vi "Config Power Sequence.vi"(7 "Get/Update":enum16{"Get Seq", "Update Seq"}(ring), 8 "Error In":errorcluster, 10 "Power Seq":T1 {"Duration" format="%<%H:%M:%S>t"}, 11 "Seq file path":path=path "C:/Users/skkjh/OneDrive - Chroma ATE/Working Copy/Cobra Single/NI-9651 SoM RT/RT_Configuration file/Cobra Extra Settings.ini") -> (0 "Error Out":errorcluster, 2 "Power Seq out":T1 {"Duration" format="%<%H:%M:%S>t"}, 3 "Seq path out":path)   [LabVIEW 2019, in "GUI.lvlib"]
uses:
  GUI.lvlib
  Controls/Profile Sequence.ctl
  <vilib>/Utility/config.llb/Read Key (I32).vi
  <vilib>/Utility/config.llb/Read Key (U32).vi
  <vilib>/Utility/config.llb/Read Key (String).vi
  <vilib>/Utility/config.llb/Write Key (String).vi
  <vilib>/Utility/config.llb/Write Key (I32).vi
  <vilib>/Utility/config.llb/Write Key (Double).vi
  <vilib>/Utility/config.llb/NI_LVConfig.lvlib
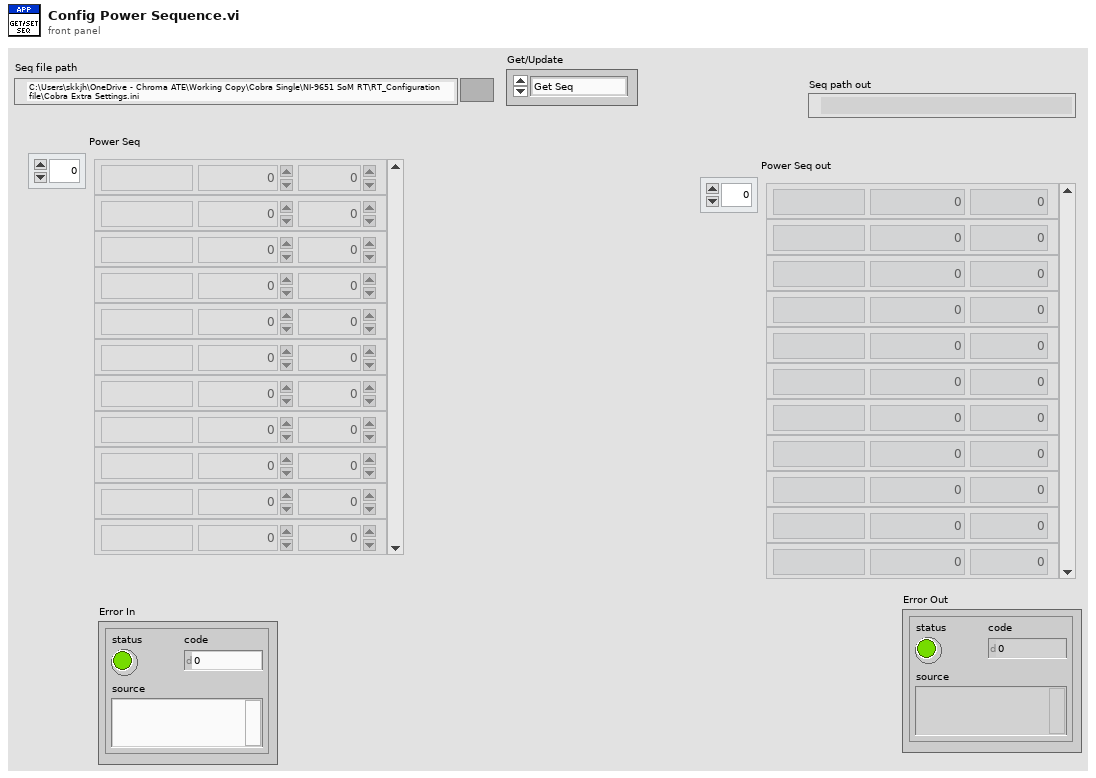
[diagram p1: front panel]
types:
  T1 = typedef "GUI.lvlib/Profile Sequence.ctl" = cluster{"Duration":i32, "Head Load(W)":u32, "Name":string}[]
  T2 = typedef "NI_LVConfig.lvlib/Config Data RefNum.ctl" = refnum<k1>
  T3 = cluster{"Duration":i32, "Head Load(W)":u32, "Name":string}
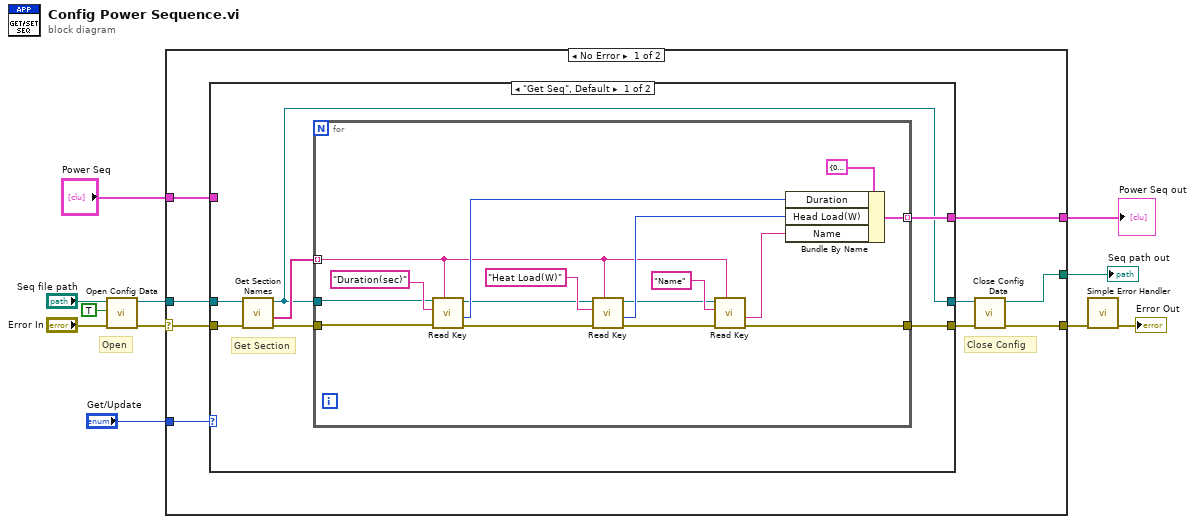
[diagram p0: block diagram]
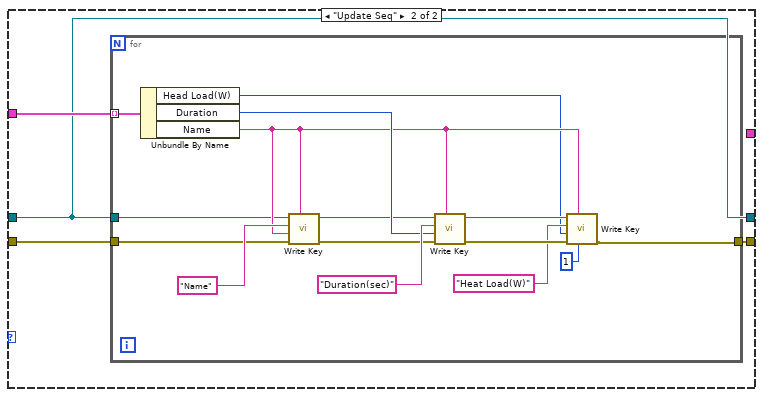
[diagram p2: hidden frame]
diagram:
  # "Open"
  n1 = call <vilib>:"Open Config Data.vi"("error in (no error)"="Error In", "create file if necessary (T)"=TRUE, "configuration file path"="Seq file path") -> ("error out"=w7:errorcluster, "refnum"=w6:T2)  [unwired: 6 in, 1 out]
  n2 = case shown="No Error" w7 {
    selector: w7 -> [w15 w63]
    tunnel: "Get/Update" -> [w20 _]
    tunnel: [w17 w63] -> w10
    tunnel: "Power Seq" -> [w18 _]
    tunnel: [w16 _] -> w1
    tunnel: w6 -> [w14 _]
    tunnel: [w12 _] -> w3
    frame No Error {
      # "Close Config"
      n3 = case shown="\"Get Seq\", Default" w20 {
        tunnel: w15 -> [w23 w45]
        tunnel: [w27 w46] -> w19
        tunnel: [w21 w44] -> w13
        tunnel: w18 -> [_ w47]
        tunnel: [w26 _] -> w16
        tunnel: w14 -> [w22 w44]
        frame "Get Seq", Default {
          # "Get Section"
          n4 = call <vilib>:"Get Section Names.vi"("error in (no error)"=w23, "refnum"=w22) -> ("error out"=w25:errorcluster, "section names"=w24:string[], "refnum out"=w21:T2)  [unwired: 7 in]
          n5 = for {
            tunnel: w25 -> [w31]
            tunnel: w21 -> [w32]
            tunnel: w24 -> [w33] mode=indexing
            tunnel: [w35] -> w27
            tunnel: [w41] -> w26 mode=indexing
            n6 = call-poly <vilib>:"Read Key.vi"("section"=w33, "error in (no error)"=w31, "key"="Duration(sec)", "refnum"=w32) -> ("error out"=w39:errorcluster, "value"=w42:i32, "refnum out"=w37:T2)  [unwired: 4 in, 1 out]
            n7 = call-poly <vilib>:"Read Key.vi"("section"=w33, "error in (no error)"=w39, "key"="Heat Load(W)", "refnum"=w37) -> ("error out"=w28:errorcluster, "value"=w38:u32, "refnum out"=w29:T2)  [unwired: 4 in, 1 out]
            n8 = call-poly <vilib>:"Read Key.vi"("section"=w33, "error in (no error)"=w28, "key"="Name", "refnum"=w29) -> ("error out"=w35:errorcluster, "value"=w34:string)  [unwired: 4 in, 2 out]
            n9 = Bundle By Name(cluster=T3 {"Duration"=0, "Head Load(W)"=0, "Name"=""} ("Sequence"), "Duration"=w42, "Head Load(W)"=w38, "Name"=w34) -> (w41:T3)
          }
        }
        frame "Update Seq" {
          n10 = for {
            tunnel: w47 -> [w61] mode=indexing
            tunnel: w45 -> [w52]
            tunnel: w44 -> [w51]
            tunnel: [w49] -> w46
            n11 = Unbundle By Name(w61) -> ("Head Load(W)"=w48:u32, "Duration"=w60:i32, "Name"=w54:string)
            n12 = call-poly <vilib>:"Write Key.vi"("section"=w54, "error in (no error)"=w52, "value"=w54, "key"="Name", "refnum"=w51) -> ("error out"=w57:errorcluster, "refnum out"=w55:T2)  [unwired: 4 in, 1 out]
            n13 = call-poly <vilib>:"Write Key.vi"("section"=w54, "error in (no error)"=w57, "value"=w60, "key"="Duration(sec)", "refnum"=w55) -> ("error out"=w59:errorcluster, "refnum out"=w58:T2)  [unwired: 4 in, 1 out]
            n14 = call-poly <vilib>:"Write Key.vi"("precision (6)"=i16 1, "section"=w54, "error in (no error)"=w59, "value"=w48, "key"="Heat Load(W)", "refnum"=w58) -> ("error out"=w49:errorcluster)  [unwired: 3 in, 2 out]
          }
        }
      }
      n15 = call <vilib>:"Close Config Data.vi"("error in (no error)"=w19, "refnum"=w13) -> ("error out"=w17:errorcluster, "file path"=w12:path)  [unwired: 8 in]
    }
    frame Error {
    }
  }
  "Seq path out" <- w3
  "Power Seq out" <- w1
  n16 = call <vilib>:"Simple Error Handler.vi"("error in (no error)"=w10) -> ("error out"=→"Error Out":errorcluster)  [unwired: 4 in, 4 out]
